vi "GMLAN ReadUUDTResponses.vi"(8 "error in":errorcluster, 11 "UUDT Engine":T5) -> (0 "error out":errorcluster, 3 "Data":T1[](array[typedef]) {"Data"."payload" format="%x"; "Data"."timestamp" format="%<%.7X\n%x>T"; "Data"."type" items=["CAN Data"=0, "CAN Remote"=1, "CAN Bus Error"=2, "CAN 2.0 Data"=8, "CAN FD Data"=16, "CAN FD+BRS Data"=24, "J1939 Data"=192, "Delay"=224, "Log Trigger"=225, "Start Trigger"=226]; "Data"."identifier" format="%x"})   [LabVIEW 2019, in "GMLAN.lvlib"]
uses:
  GMLAN.lvlib
  _SubVIs/UUDT Engine Refs.ctl
  _SubVIs/UUDT Messages.ctl
  _SubVIs/UUDT Responses.ctl
  <vilib>/xnet/xnet.llb/XNET Frame CAN.ctl
  <vilib>/xnet/xnet.llb/XNET Frame Type CAN.ctl
  _SubVIs/UUDT Engine Connection List_Action.ctl
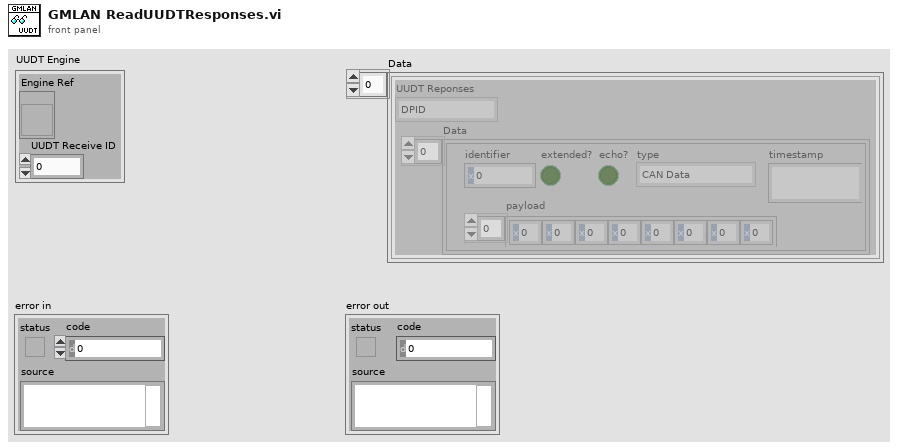
[diagram p1: front panel]
types:
  T1 = typedef "GMLAN.lvlib/UUDT Messages.ctl" = cluster{"UUDT Reponses":T2, "Data":T3[]}
  T2 = typedef "GMLAN.lvlib/UUDT Responses.ctl" = enum16{"DPID", "DTCStatus", "DTCReport", "ChangeDTCCount"}
  T3 = typedef "XNET Frame CAN.ctl" = cluster{"timestamp":timestamp, "payload":u8[], "identifier":u32, "type":T4, "extended?":bool, "echo?":bool}
  T4 = typedef "XNET Frame Type CAN.ctl" = u8
  T5 = typedef "GMLAN.lvlib/UUDT Engine Refs.ctl" = cluster{"Engine Ref":refnum<vi>, "UUDT Receive ID":u32}
  T6 = typedef "GMLAN.lvlib/UUDT Engine Connection List_Action.ctl" = enum8{"Initialize", "Write", "Add", "Read"}
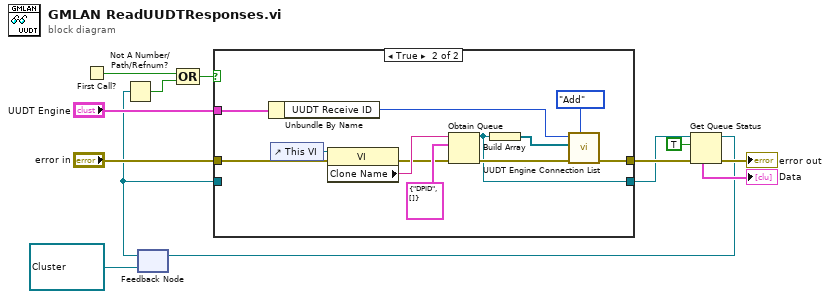
[diagram p0: block diagram]
diagram:
  n1 = First Call?() -> (First Call?: T/F=w12:bool)
  n2 = feedback #1(refnum<queue> refnum ("queue out")) -> (w9:refnum<queue>)
  n3 = Not A Number/Path/Refnum?(number/path/refnum=w9) -> (NaN/Path/Refnum?=w8:bool)
  n4 = Compound Arithmetic op=OR(w12, w8) -> (w10:bool)
  n5 = case shown="True" w10 {
    tunnel: "UUDT Engine" -> [_ w17]
    tunnel: [w15 w18] -> w4
    tunnel: w9 -> [w15 _]
    tunnel: [w14 w20] -> w6
    tunnel: "error in" -> [w14 w19]
    frame False {
    }
    frame True {
      n6 = Unbundle By Name(w17) -> ("UUDT Receive ID"=w16:u32)
      n7 = control-ref of="This VI"() -> (w27:refnum<vi>)
      n8 = property class="VI"(reference=w27, error in=w19) -> (error out=w24:errorcluster, "Clone Name"=w26:string)  [unwired: 1 out]
      n9 = Obtain Queue(name (unnamed)=w26, element data type=T1 {"UUDT Reponses"=enum."DPID", "Data"=[]} ("Cluster"), error in (no error)=w24) -> (queue out=w18:refnum<queue>, error out=w23:errorcluster)  [unwired: 2 in, 1 out]
      n10 = Build Array(w18) -> (w21:refnum<queue>[])
      n11 = call "UUDT Engine Connection List.vi"("Action"=UUDT_Engine_Connection_List_Action."Add", "error in"=w23, "Queue List"=w21, "UUDT"=w16) -> ("error out"=w20:errorcluster)  [unwired: 6 in, 1 out]
    }
  }
  n12 = Get Queue Status(queue=w4, return elements? (F)=TRUE, error in (no error)=w6) -> (queue out=w1:refnum<queue>, error out=→"error out":errorcluster, elements=→"Data":T1[])  [unwired: 5 out]
  n13 = feedback-in #1(w1) -> ()
